vi "Test Get Debug Log Filtered by Is Receive.vi"(8 "error in (no error)":errorcluster, 11 "Test Case In":refnum<class "Debugger Test.lvclass">) -> (0 "error out":errorcluster, 3 "Test Case Out":refnum<class "Debugger Test.lvclass">)   [LabVIEW 2020, in "Debugger Test.lvclass"]
uses:
  Debugger Test.lvclass
  C:/Program Files (x86)/National Instruments/LabVIEW 2020/vi.lib/Astemes/LUnit/Test Case.lvclass
  source/Debugger/Debugger.lvclass
  C:/Users/anton/Documents/GitHub/triarc-debugger/source/Process/Debug Process.lvclass
  source/Debug Data/Raw Debug Data.ctl
  source/Debug Data/Debug Data.lvclass/Debug Data.ctl
  source/Process/Debug Process.lvclass/Debug Process.ctl
  <vilib>/Astemes/LUnit/Test Case.lvclass/Test Case.ctl
  <vilib>/Astemes/LUnit/LUnit Assertion Result.lvclass/LUnit Assertion Result.ctl
  <vilib>/Astemes/LUnit/LUnit Test Case Result.lvclass/LUnit Test Case Result.ctl
  <vilib>/Astemes/LUnit/LUnit Method Result.lvclass/LUnit Method Result.ctl
  01074fa8-ee8a-411d-bc8b-fc92c4f90959.vi
  <vilib>/AdvancedString/Delimited String to 1D String Array.vi
  source/Process/Public/Lifecycle/Get Lifecycle State.vi
  <vilib>/Astemes/Triarc Framework/Broadcast Event Helpers/Execution timer.vi
  source/Process/Private/SubVIs/Wait for finish.vi
  source/Process/Protected/Messaging/Enqueue Message.vi
  source/Process/Private/SubVIs/Set Lifecycle State.vi
  <vilib>/Astemes/LUnit/Palette/Pass.vi
  <vilib>/Astemes/LUnit/Palette/Fail.vi
  <vilib>/Astemes/LUnit/Compare Variants.vi
  <vilib>/Astemes/LUnit/Describe Comparison.vi
  <vilib>/Astemes/LUnit/Set Assertion Type.vi
  <vilib>/Utility/error.llb/Clear Errors.vi
  <vilib>/Astemes/LUnit/Add test result.vi
  <vilib>/Astemes/LUnit/LUnit Write Passed.vi
  <vilib>/Astemes/LUnit/LUnit Write Message.vi
  <vilib>/Astemes/LUnit/LUnit Write Description.vi
  <vilib>/Astemes/LUnit/Variant to string.vi
  <vilib>/Astemes/LUnit/LUnit Write Assertion Type.vi
  <vilib>/Astemes/LUnit/LUnit Record Assertion Result.vi
  <vilib>/Astemes/LUnit/LUnit Aggregate Assertion Results.vi
  <vilib>/Astemes/LUnit/Assertion Result/LUnit Read Status.vi
  <vilib>/Astemes/LUnit/LUnit Read Message.vi
  <vilib>/Astemes/LUnit/LUnit Read Description.vi
  <vilib>/Astemes/LUnit/Method Result/LUnit Merge Status.vi
  <vilib>/Astemes/LUnit/LUnit Concatenate result strings.vi
  <vilib>/Utility/error.llb/Error Cluster From Error Code.vi
  <vilib>/Astemes/Triarc Framework/Broadcast Event Helpers/Dequeue Broadcast Message.vi
  <vilib>/Utility/Data Type/Get Type Information.vi
  <vilib>/Utility/LVClass/Get LV Class Name.vi
  source/Debug Data/Debug Data.lvclass
  <vilib>/Astemes/LUnit/LUnit Assertion Result.lvclass
  source/Process/Debug Process.lvclass
  <vilib>/Astemes/Triarc Framework/Broadcast Event Helpers/Broadcast Event Helpers.lvlib
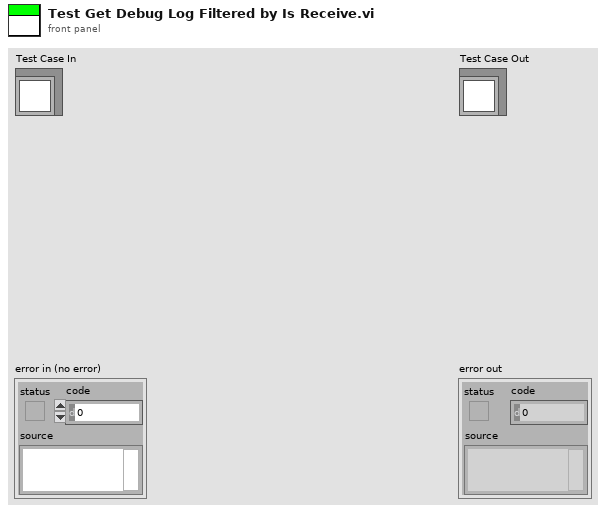
[diagram p1: front panel]
types:
  T1 = typedef "Debug Data.lvclass/Raw Debug Data.ctl" = cluster{"Action":string, "Call Chain":string, "Process":string, "Message":string, "Message Data":variant, "Time":dbl}
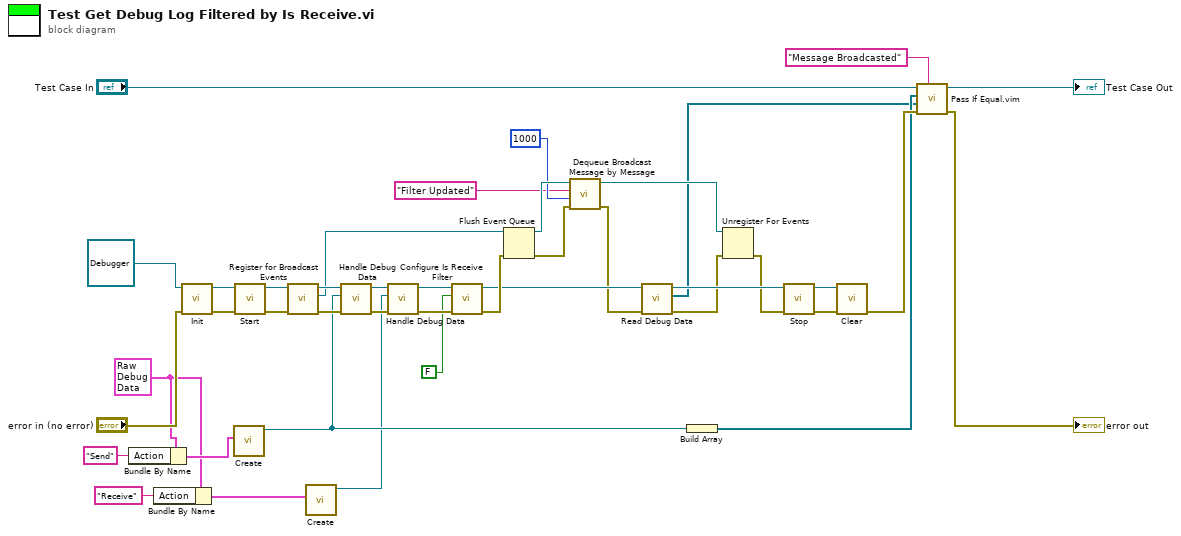
[diagram p0: block diagram]
diagram:
  w14 = T1 {"Action"="", "Call Chain"="", "Process"="", "Message"="", "Message Data"=variant, "Time"=0.0} ("Debug Data Cluster")
  n1 = Bundle By Name(cluster=w14, "Action"="Send" ("Process")) -> (w22:T1)
  n2 = Bundle By Name(cluster=w14, "Action"="Receive" ("Process")) -> (w15:T1)
  n3 = call-dynamic "Init.vi"("error in (no error)"="error in (no error)", "Process In"=refnum<class "Debugger.lvclass"> refnum ("Debug Data Event In 2")) -> ("error out"=w37:errorcluster, "Process Out"=w38:refnum<class "Debugger.lvclass">)  [unwired: 8 in]
  n4 = call "Create.vi"("Debug Data Cluster"=w22) -> ("Debug Data out"=w25:refnum<class "Debug Data.lvclass">)  [unwired: 9 in, 1 out]
  n5 = call "Start.vi"("error in (no error)"=w37, "Process In"=w38) -> ("error out"=w35:errorcluster, "Process Out"=w36:refnum<class "Debugger.lvclass">)  [unwired: 7 in, 1 out]
  n6 = call "Register for Broadcast Events.vi"("error in (no error)"=w35, "Process In"=w36) -> ("error out"=w34:errorcluster, "Event Registration Refnum Out"=w23:refnum<event-registration>, "Process Out"=w30:refnum<class "Debugger.lvclass">)  [unwired: 7 in]
  n7 = call "Create.vi"("Debug Data Cluster"=w15) -> ("Debug Data out"=w17:refnum<class "Debug Data.lvclass">)  [unwired: 9 in, 1 out]
  n8 = call-dynamic "Handle Debug Data.vi"("error in (no error)"=w34, "Debug Data.lvclass"=w25, "Debug Data Event In"=w30) -> ("error out"=w19:errorcluster, "Debug Data Event Out"=w20:refnum<class "Debugger.lvclass">)  [unwired: 7 in]
  n9 = call-dynamic "Handle Debug Data.vi"("error in (no error)"=w19, "Debug Data.lvclass"=w17, "Debug Data Event In"=w20) -> ("error out"=w18:errorcluster, "Debug Data Event Out"=w12:refnum<class "Debugger.lvclass">)  [unwired: 7 in]
  n10 = call "Configure Is Receive Filter.vi"("error in (no error)"=w18, "Show Receive?"=FALSE ("Show Send?"), "Debugger In"=w12) -> ("error out"=w13:errorcluster, "Debugger Out"=w11:refnum<class "Debugger.lvclass">)  [unwired: 7 in]
  n11 = Flush Event Queue(0:w23, 3:w13) -> (8:w7:refnum<event-registration>, 11:w1:errorcluster)  [unwired: 4 in, 1 out]
  n12 = call <vilib>:"Dequeue Broadcast Message by Message.vi"("error in (no error)"=w1, "Timeout (-1)"=1000, "Message"="Filter Updated", "Event Registration Refnum"=w7) -> ("error out"=w2:errorcluster, "Event Registration Refnum Out"=w4:refnum<event-registration>)  [unwired: 3 in, 3 out]
  n13 = call "Read Debug Data.vi"("error in (no error)"=w2, "Debugger In"=w11) -> ("error out"=w10:errorcluster, "Data Log"=w3:refnum<class "Debug Data.lvclass">[], "Debugger Out"=w33:refnum<class "Debugger.lvclass">)  [unwired: 7 in]
  n14 = Build Array(w25) -> (w24:refnum<class "Debug Data.lvclass">[])
  n15 = Unregister For Events(event registration refnum=w4, error in=w10) -> (error out=w9:errorcluster)
  n16 = call "Stop.vi"("error in (no error)"=w9, "Process In"=w33) -> ("error out"=w31:errorcluster, "Process Out"=w32:refnum<class "Debugger.lvclass">)  [unwired: 7 in, 1 out]
  n17 = call-dynamic "Clear.vi"("error in (no error)"=w31, "Process In"=w32) -> ("error out"=w27:errorcluster)  [unwired: 9 in]
  n18 = call "Pass If Equal.vim"("Description"="Message Broadcasted", "error in (no error)"=w27, "Actual"=w3, "Expected"=w24, "LUnit Test Case In"="Test Case In") -> ("error out"=→"error out":errorcluster, "LUnit Test Case Out"=→"Test Case Out":refnum<class "Debugger Test.lvclass">)  [unwired: 5 in]
